vi "piezoWriteUSBClose.vi"   [LabVIEW 2017]
uses:
  Piezo/lvlib/Madlib.lvlib
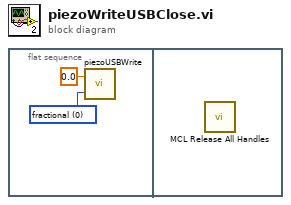
[diagram p0: block diagram]
diagram:
  n1 = flat-sequence {
    frame #0 {
      w1 = u16 0 items=["fractional", "voltage (V)", "position (um)"] ("mode")
      n2 = call "piezoUSBWrite.vi"("mode"=w1, "position"=0.0) -> ()  [unwired: 1 in]
    }
    frame #1 {
      n3 = call "MCL Release All Handles.vi"() -> ()  [unwired: 12 in]
    }
  }
